vi "Function.vi"(8 "error in (no error)":errorcluster, 9 "Numeric":dbl, 10 "Waveform":waveform(dbl), 11 "Two Terminal in":refnum<class "Add_WFM_Numeric.lvclass">) -> (0 "error out":errorcluster, 2 "Result":waveform(dbl), 3 "Two Terminal out":refnum<class "Add_WFM_Numeric.lvclass">)   [LabVIEW 2021, in "Add_WFM_Numeric.lvclass"]
uses:
  Add_WFM_Numeric.lvclass
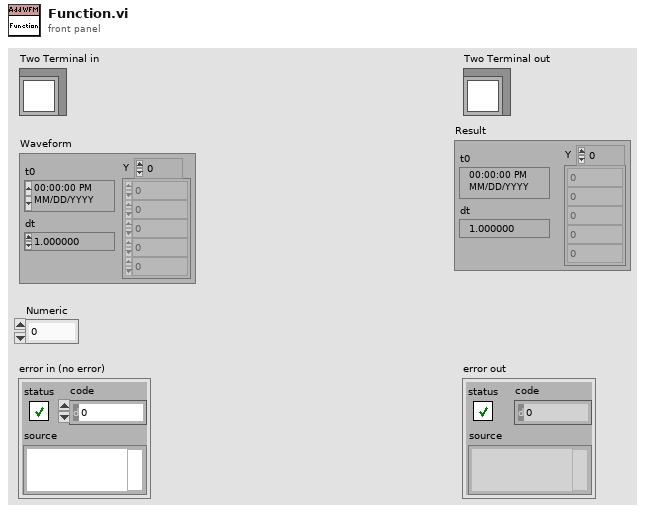
[diagram p1: front panel]
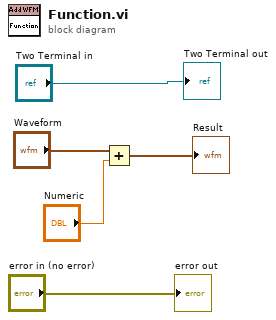
[diagram p0: block diagram]
diagram:
  n1 = Add(x="Waveform", y="Numeric") -> (x+y=→"Result":waveform(dbl))
  "error out" <- "error in (no error)"
  "Two Terminal out" <- "Two Terminal in"
